vi "Read Image Type.vi"() -> (3 "Output Image Type":T1)   [LabVIEW 2020, in "SimpleDependencyInspector.lvlib"]
uses:
  SimpleDependencyInspector.lvlib
  Image Type--enum.ctl
  <resource>/dialog/lvconfig.llb/LV Config Read Numeric (I32).vi
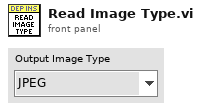
[diagram p1: front panel]
types:
  T1 = typedef "SimpleDependencyInspector.lvlib/Image Type--enum.ctl" = enum16{"JPEG", "PNG", "BMP", "SVG"}
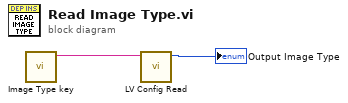
[diagram p0: block diagram]
diagram:
  n1 = call "Image Type key.vi"() -> ("String"=w2:string)  [unwired: 11 in]
  n2 = call-poly <resource>:"LV Config Read.vi"("key"=w2) -> ("value"=→"Output Image Type":i32)  [unwired: 4 in, 2 out]
